vi "esp32.vi"() -> ()   [LabVIEW 2017]
panel:
  out "parameter value":string
  out "function value":string
  in  "stop 4":bool
  out "NewVal":enum16{"input", "output", "disable"}(ring)
  out "appended array":refnum<vi>[](array[refnum])
  out "bytes written 4":i32
  out "bytes written 2":i32
  in  "stop 3":bool
  in  "Tab Control":T1(tab)
  in  "address":string="10.5.4.109"
  in  "Port":u16=8888
  in  "pin 14":enum16{"input", "output", "disable"}(ring)=enum."disable"
  in  "VIN":enum16{""}(ring)
  in  "GND 2":enum16{""}(ring)
  in  "3.3 V":enum16{""}(ring)
  in  "GND":enum16{""}(ring)
  in  "pin 15":enum16{"input", "output", "disable"}(ring)=enum."disable"
  in  "pin 02":enum16{"input", "output", "disable"}(ring)=enum."disable"
  in  "pin 04":enum16{"input", "output", "disable"}(ring)=enum."disable"
  in  "pin 16":enum16{"input", "output", "disable"}(ring)=enum."disable"
  in  "pin 17":enum16{"input", "output", "disable"}(ring)=enum."disable"
  in  "pin 05":enum16{"input", "output", "disable"}(ring)=enum."disable"
  in  "pin 18":enum16{"input", "output", "disable"}(ring)=enum."disable"
  in  "pin 19":enum16{"input", "output", "disable"}(ring)=enum."disable"
  in  "pin 21":enum16{"input", "output", "disable"}(ring)=enum."disable"
  in  "pin 03":enum16{"input", "output", "disable"}(ring)=enum."disable"
  in  "pin 01":enum16{"input", "output", "disable"}(ring)=enum."disable"
  in  "pin 22":enum16{"input", "output", "disable"}(ring)=enum."disable"
  in  "pin 23":enum16{"input", "output", "disable"}(ring)=enum."disable"
  in  "pin 12":enum16{"input", "output", "disable"}(ring)=enum."disable"
  in  "pin 27":enum16{"input", "output", "disable"}(ring)=enum."disable"
  in  "pin 26":enum16{"input", "output", "disable"}(ring)=enum."disable"
  in  "pin 25":enum16{"input", "output", "disable"}(ring)=enum."disable"
  in  "pin 33":enum16{"input", "output", "disable"}(ring)=enum."disable"
  in  "pin 32":enum16{"input", "output", "disable"}(ring)=enum."disable"
  in  "pin 35":enum16{"input", "output", "disable"}(ring)=enum."disable"
  in  "pin 34":enum16{"input", "output", "disable"}(ring)=enum."disable"
  in  "pin 39":enum16{"input", "output", "disable"}(ring)=enum."disable"
  in  "pin 36":enum16{"input", "output", "disable"}(ring)=enum."disable"
  in  "EN":enum16{""}(ring)
  in  "pin 13":enum16{"disable", "input", "output"}(ring)
  in  "output 36":bool
  out "input 36":bool
  in  "output 39":bool
  out "input 39":bool
  in  "output 12":bool
  in  "output 15":bool
  out "input 15":bool
  in  "output 2":bool
  out "input 2":bool
  in  "output 4":bool
  out "input 4":bool
  in  "output 16":bool
  out "input 16":bool
  in  "output 17":bool
  out "input 17":bool
  in  "output 5":bool
  out "input 5":bool
  in  "output 18":bool
  out "input 18":bool
  in  "output 19":bool
  out "input 19":bool
  in  "output 21":bool
  out "input 21":bool
  in  "output 3":bool
  out "input 3":bool
  in  "output 1":bool
  out "input 1":bool
  in  "output 22":bool
  out "input 22":bool
  in  "output 23":bool
  out "input 23":bool
  in  "output 34":bool
  out "input 34":bool
  out "input 13":bool
  in  "output 35":bool
  out "input 35":bool
  in  "output 32":bool
  out "input 32":bool
  in  "output 33":bool
  out "input 33":bool
  in  "output 25":bool
  out "input 25":bool
  in  "output 26":bool
  out "input 26":bool
  in  "output 27":bool
  out "input 27":bool
  in  "output 14":bool
  out "input 14":bool
  in  "output 13":bool
  out "input 12":bool
  in  "data in":string
  in  "Send Button":bool
  in  "stop 2":bool
  out "bytes written 3":i32
  out "data out":string
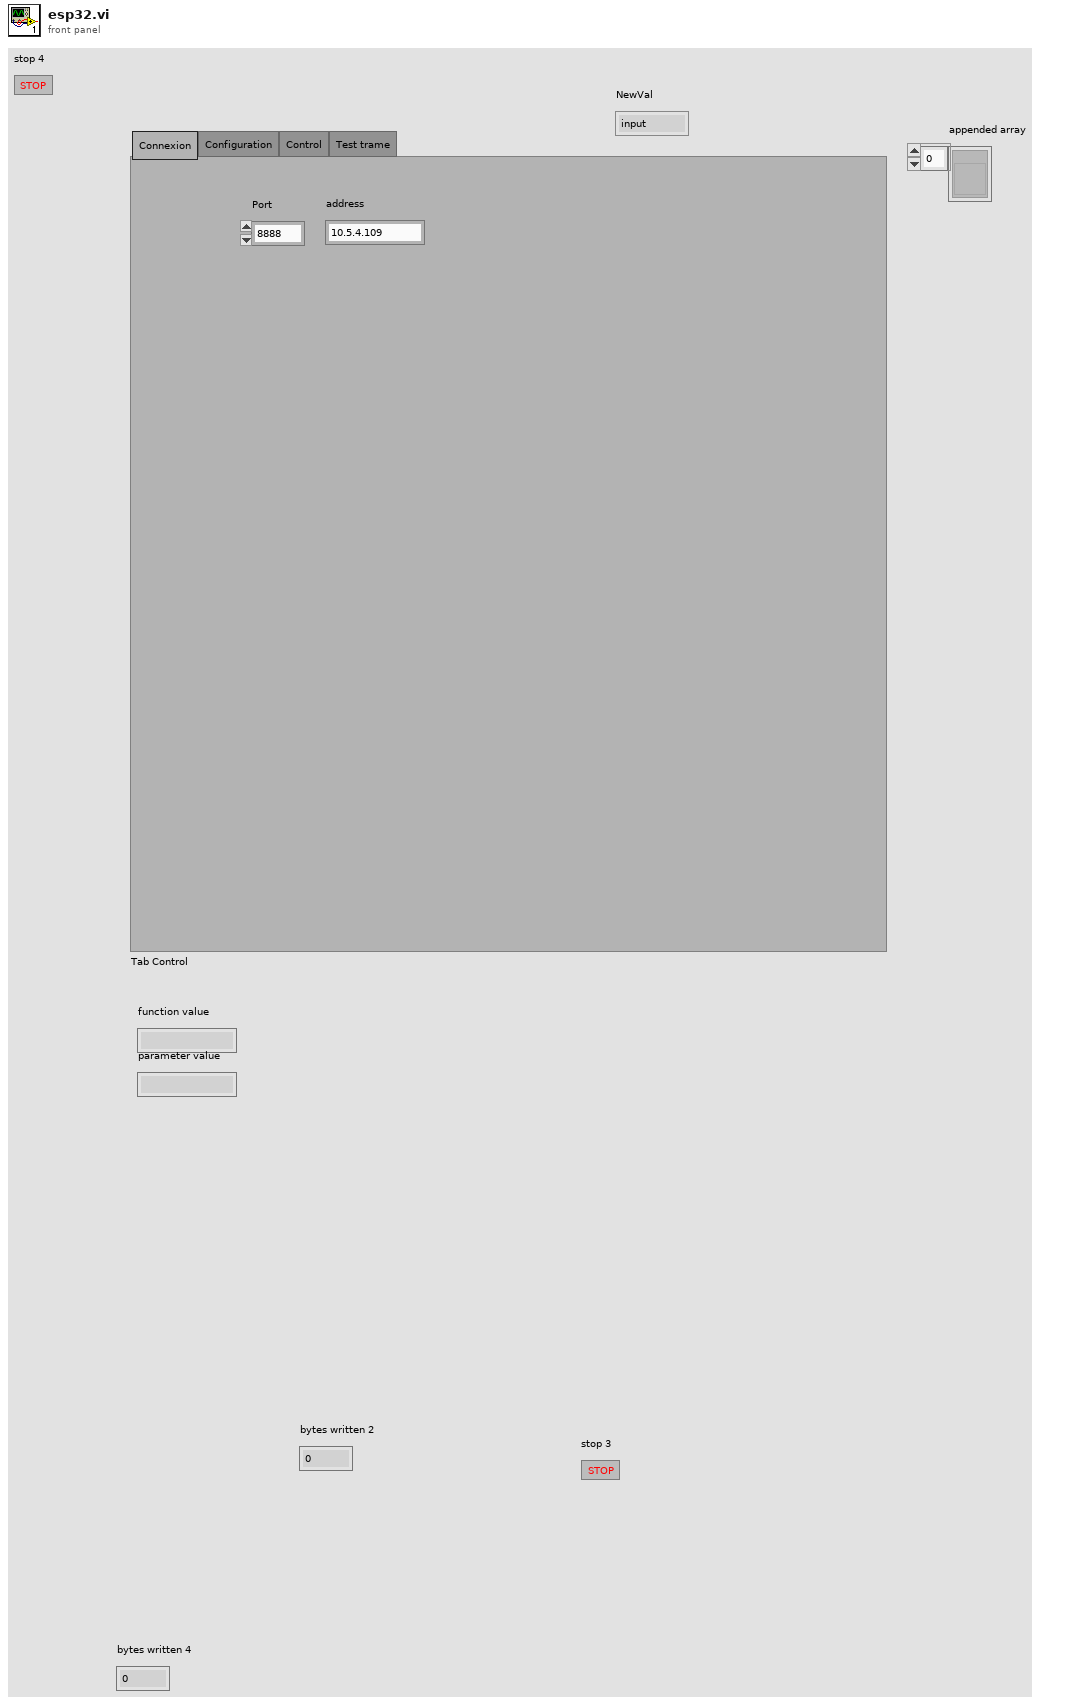
[diagram p1: front panel]
types:
  T1 = enum32{"Connexion", "Configuration", "Control", "Test trame"}
  T2 = enum16{"Standard", "Buffered", "CRLF", "Immediate"}
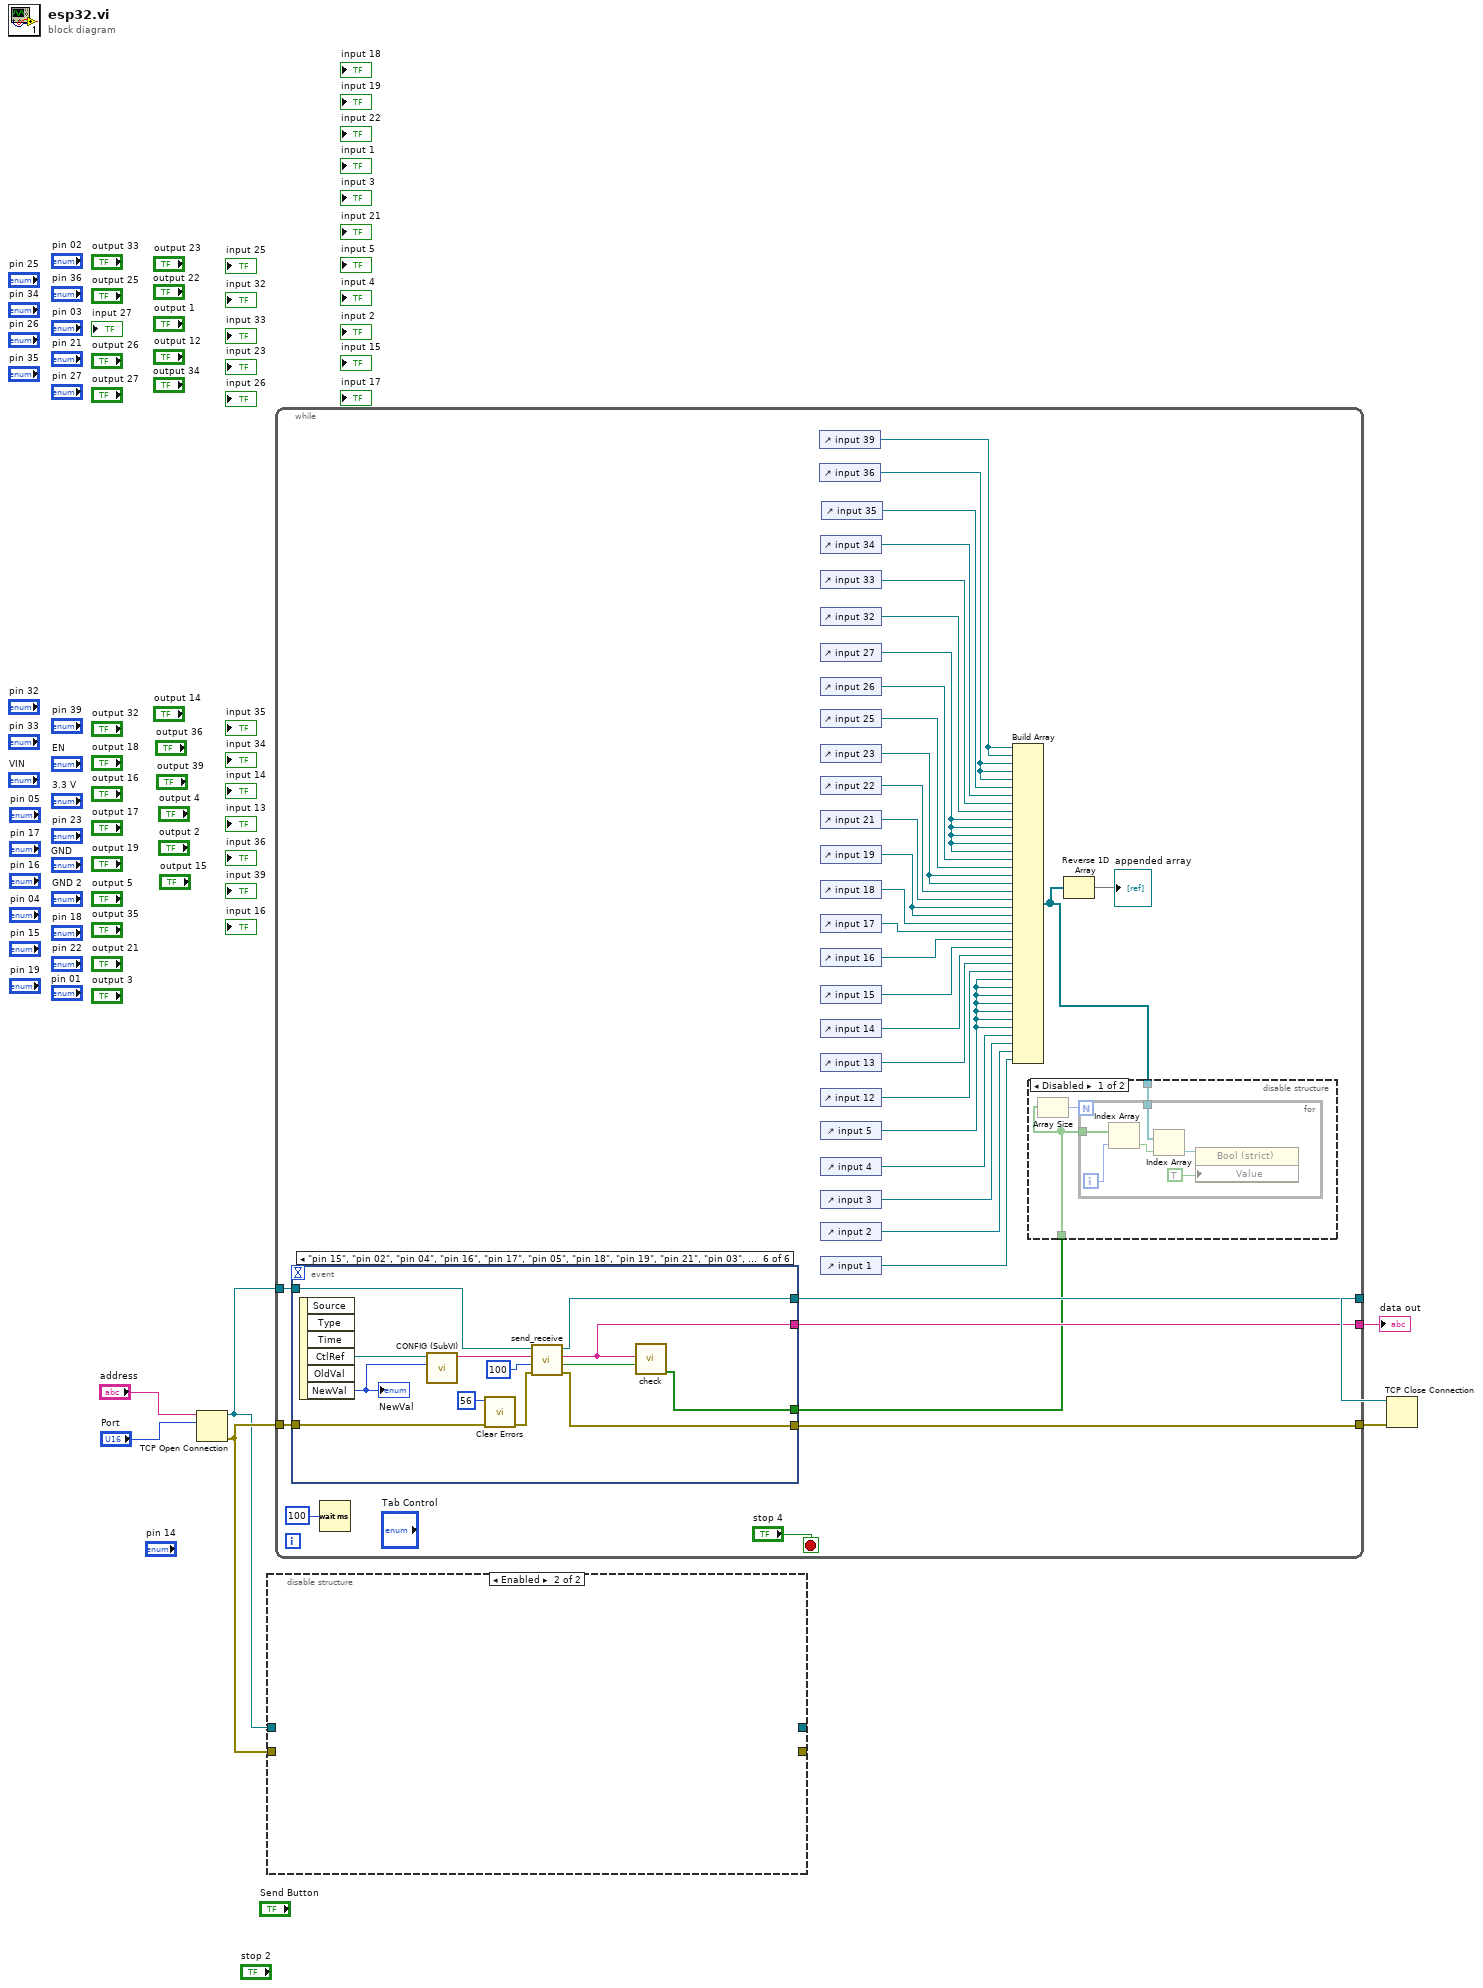
[diagram p0: block diagram]
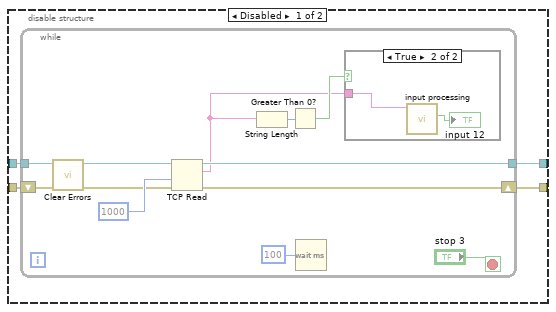
[diagram p2: hidden frame]
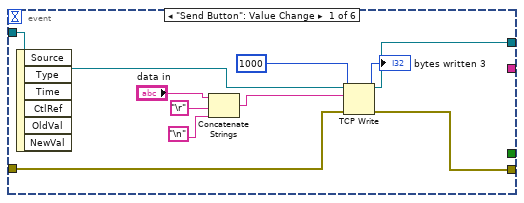
[diagram p5: hidden frame]
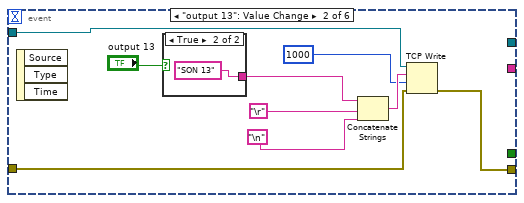
[diagram p6: hidden frame]
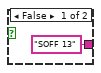
[diagram p7: hidden frame]
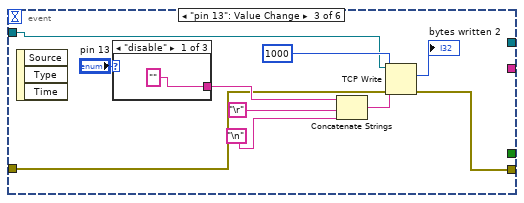
[diagram p8: hidden frame]
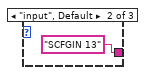
[diagram p9: hidden frame]
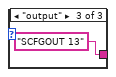
[diagram p10: hidden frame]
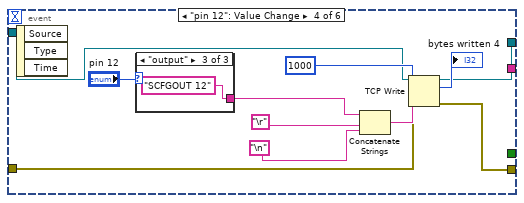
[diagram p11: hidden frame]
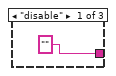
[diagram p12: hidden frame]
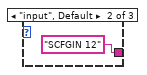
[diagram p13: hidden frame]
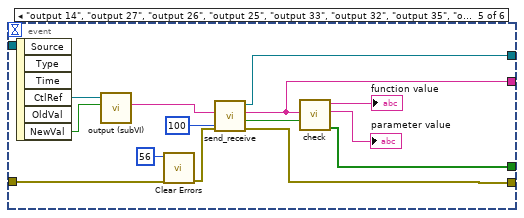
[diagram p14: hidden frame]
diagram:
  n1 = TCP Open Connection(address="address", remote port or service name="Port") -> (connection ID=w4:refnum<k5>, error out=w5:errorcluster)  [unwired: 3 in]
  n2 = disable-structure shown="Enabled" {
    disable-tunnel: w5 -> [w11 _]
    disable-tunnel: w4 -> [w10 _]
    disable-tunnel: [w9 _] -> _
    disable-tunnel: [w8 _] -> _
    frame Disabled {
      n3 = while {
        tunnel: w10 -> [w24]
        shift-right: [w22] -> w9
        shift-left: w11 -> [w18]
        tunnel: [w21] -> w8
        stop <- "stop 3" stop-if-true
        n4 = call <vilib>:"Clear Errors.vi"("error in (no error)"=w18) -> ("error out"=w17:errorcluster)  [unwired: 5 in, 1 out]
        n5 = TCP Read(connection ID=w24, error in (no error)=w17, 9:1000 ("timeout ms (25000)")) -> (bytes to read=w13:i32, connection ID out=w21:refnum<k5>, data out=w14:string, error out=w22:errorcluster, 7:w12:T2)
        n6 = String Length(string=w14) -> (length=w16:i32)
        n7 = Greater Than 0?(x=w16) -> (x > 0?=w15:bool)
        n8 = Wait (ms)(milliseconds to wait=u32 100) -> ()  [unwired: 1 out]
        n9 = case shown="True" w15 {
          tunnel: w14 -> [_ w25]
          frame False {
          }
          frame True {
            n10 = call "input processing.vi"("String"=w25) -> ("inputan 5"=→"input 12":bool)  [unwired: 9 in, 1 out]
          }
        }
      }
    }
    frame Enabled {
    }
  }
  n11 = while {
    tunnel: w5 -> [w60]
    tunnel: [w58] -> w2
    tunnel: w4 -> [w61]
    tunnel: [w57] -> w1
    tunnel: [w55] -> w3
    stop <- "stop 4" stop-if-true
    n12 = event shown="[5] \"pin 15\", \"pin 02\", \"pin 04\", \"pin 16\", \"pin 17\", \"pin 05\", \"pin 18\", \"pin 19\", \"pin 21\", \"pin 03\", \"pin 01\", \"pin 22\", \"pin 23\", \"pin 27\", \"pin 26\", \"pin 25\", \"pin 33\", \"pin 32\", \"pin 35\", \"pin 34\", \"pin 39\", \"pin 36\", \"pin 14\": Value Change" {
      selector: _ -> [_ _ _ _ _ _]
      dyn-events: _ -> [_ _ _ _ _ _]
      timeout: _ -> [_ _ _ _ _ _]
      tunnel: w61 -> [w73 w81 w92 w106 _ w142]
      tunnel: w60 -> [w75 w82 w93 w107 w127 w137]
      tunnel: [w74 w84 w94 w108 w128 w138] -> w58
      tunnel: [w72 _ _ w105 w123 w139] -> w57
      tunnel: [_ _ _ _ w122 w134] -> w55
      tunnel: [_ _ _ _ w119 w133] -> w27
      event "Send Button": Value Change {
        n13 = event-data() -> ()  [unwired: 1 in, 6 out]
        n14 = Concatenate Strings("data in", "\r", "\n") -> (w80:string)
        n15 = TCP Write(connection ID=w73, data in=w80, error in (no error)=w75, 9:1000 ("timeout ms (25000)")) -> (connection ID out=w72:refnum<k5>, bytes written=→"bytes written 3":i32, error out=w74:errorcluster)
      }
      event "output 13": Value Change {
        n16 = event-data() -> ()  [unwired: 1 in, 3 out]
        n17 = case shown="True" "output 13" {
          tunnel: ["SOFF 13" "SON 13"] -> w83
          frame False {
          }
          frame True {
          }
        }
        n18 = Concatenate Strings(w83, "\r", "\n") -> (w88:string)
        n19 = TCP Write(connection ID=w81, data in=w88, error in (no error)=w82, 9:1000 ("timeout ms (25000)")) -> (error out=w84:errorcluster)  [unwired: 2 out]
      }
      event "pin 13": Value Change {
        n20 = event-data() -> ()  [unwired: 1 in, 3 out]
        n21 = case shown="\"disable\"" "pin 13" {
          tunnel: ["" "SCFGIN 13" "SCFGOUT 13"] -> w95
          frame "disable" {
          }
          frame "input", Default {
          }
          frame "output" {
          }
        }
        n22 = Concatenate Strings(w95, "\r", "\n") -> (w100:string)
        n23 = TCP Write(connection ID=w92, data in=w100, error in (no error)=w93, 9:1000 ("timeout ms (25000)")) -> (bytes written=→"bytes written 2":i32, error out=w94:errorcluster)  [unwired: 1 out]
      }
      event "pin 12": Value Change {
        n24 = event-data() -> ()  [unwired: 1 in, 3 out]
        n25 = case shown="\"output\"" "pin 12" {
          tunnel: ["" "SCFGIN 12" "SCFGOUT 12"] -> w110
          frame "disable" {
          }
          frame "input", Default {
          }
          frame "output" {
          }
        }
        n26 = Concatenate Strings(w110, "\r", "\n") -> (w115:string)
        n27 = TCP Write(connection ID=w106, data in=w115, error in (no error)=w107, 9:1000 ("timeout ms (25000)")) -> (connection ID out=w105:refnum<k5>, bytes written=→"bytes written 4":i32, error out=w108:errorcluster)
      }
      event "output 14", "output 27", "output 26", "output 25", "output 33", "output 32", "output 35", "output 34", "output 23", "output 22", "output 1", "output 3", "output 21", "output 19", "output 18", "output 5", "output 17", "output 16", "output 4", "output 2", "output 15", "output 12", "output 39", "output 36": Value Change {
        n28 = event-data() -> ("CtlRef"=w125:refnum<vi>, "NewVal"=w126:bool)  [unwired: 1 in, 4 out]
        n29 = call "output (subVI).vi"("NewVal in"=w126, "Boolean in"=w125) -> ("string out"=w124:string)  [unwired: 9 in]
        n30 = call <vilib>:"Clear Errors.vi"("error in (no error)"=w127, "specific error code to clear (0: all)"=56) -> ("error out"=w130:errorcluster)  [unwired: 4 in, 1 out]
        n31 = call "send_receive.vi"("error in (no error)"=w130, "time"=u32 100, "data in"=w124) -> ("error out"=w128:errorcluster, "Result"=w132:bool, "data out"=w122:string, "connection ID out"=w123:refnum<k5>)  [unwired: 5 in]
        n32 = call "check.vi"("input result"=w132, "input string"=w122) -> ("Array"=w119:bool[], "parameter value"=→"parameter value":string, "function value"=→"function value":string)  [unwired: 6 in, 1 out]
      }
      event "pin 15", "pin 02", "pin 04", "pin 16", "pin 17", "pin 05", "pin 18", "pin 19", "pin 21", "pin 03", "pin 01", "pin 22", "pin 23", "pin 27", "pin 26", "pin 25", "pin 33", "pin 32", "pin 35", "pin 34", "pin 39", "pin 36", "pin 14": Value Change {
        n33 = event-data() -> ("CtlRef"=w145:refnum<vi>, "NewVal"=w144:enum16{"input", "output", "disable"})  [unwired: 1 in, 4 out]
        "NewVal" <- w144
        n34 = call "CONFIG (SubVI).vi"("NewVal"=w144, "Enum in"=w145) -> ("String"=w143:string)  [unwired: 9 in]
        n35 = call <vilib>:"Clear Errors.vi"("error in (no error)"=w137, "specific error code to clear (0: all)"=56) -> ("error out"=w136:errorcluster)  [unwired: 4 in, 1 out]
        n36 = call "send_receive.vi"("error in (no error)"=w136, "time"=u32 100, "data in"=w143, "connection ID in"=w142) -> ("error out"=w138:errorcluster, "Result"=w141:bool, "data out"=w134:string, "connection ID out"=w139:refnum<k5>)  [unwired: 4 in]
        n37 = call "check.vi"("input result"=w141, "input string"=w134) -> ("Array"=w133:bool[])  [unwired: 6 in, 3 out]
      }
    }
    n38 = Wait (ms)(milliseconds to wait=u32 100) -> ()  [unwired: 1 out]
    n39 = control-ref of="input 39"() -> (w53:refnum<vi>)
    n40 = control-ref of="input 36"() -> (w52:refnum<vi>)
    n41 = control-ref of="input 34"() -> (w50:refnum<vi>)
    n42 = control-ref of="input 33"() -> (w49:refnum<vi>)
    n43 = control-ref of="input 32"() -> (w48:refnum<vi>)
    n44 = control-ref of="input 27"() -> (w47:refnum<vi>)
    n45 = control-ref of="input 26"() -> (w46:refnum<vi>)
    n46 = control-ref of="input 25"() -> (w45:refnum<vi>)
    n47 = control-ref of="input 23"() -> (w44:refnum<vi>)
    n48 = control-ref of="input 22"() -> (w43:refnum<vi>)
    n49 = control-ref of="input 21"() -> (w42:refnum<vi>)
    n50 = control-ref of="input 19"() -> (w41:refnum<vi>)
    n51 = control-ref of="input 18"() -> (w40:refnum<vi>)
    n52 = control-ref of="input 17"() -> (w39:refnum<vi>)
    n53 = control-ref of="input 16"() -> (w38:refnum<vi>)
    n54 = control-ref of="input 15"() -> (w37:refnum<vi>)
    n55 = control-ref of="input 14"() -> (w36:refnum<vi>)
    n56 = control-ref of="input 13"() -> (w35:refnum<vi>)
    n57 = control-ref of="input 12"() -> (w34:refnum<vi>)
    n58 = control-ref of="input 5"() -> (w33:refnum<vi>)
    n59 = control-ref of="input 4"() -> (w31:refnum<vi>)
    n60 = control-ref of="input 3"() -> (w30:refnum<vi>)
    n61 = control-ref of="input 2"() -> (w29:refnum<vi>)
    n62 = control-ref of="input 1"() -> (w32:refnum<vi>)
    n63 = control-ref of="input 35"() -> (w51:refnum<vi>)
    n64 = Build Array(w53, w53, w52, w52, w52, w51, w50, w49, w48, w47, w47, w47, w47, w47, w46, w45, w44, w44, w43, w42, w41, w41, w40, w39, w38, w37, w36, w35, w34, w33, w33, w33, w33, w33, w33, w33, w31, w30, w29, w32) -> (w28:refnum<vi>[])
    n65 = disable-structure shown="Disabled" {
      disable-tunnel: w28 -> [w64 _]
      disable-tunnel: w27 -> [w62 _]
      frame Disabled {
        n66 = Array Size(array=w62) -> (size(s)=w63:i32)
        n67 = for {
          N: w63 -> [_]
          tunnel: w62 -> [w70]
          tunnel: w64 -> [w67]
          i -> [w69]
          n68 = Index Array(array=w70, index=w69) -> (element=w66:bool)
          n69 = Index Array(array=w67, index=w66) -> (element=w68:refnum<vi>)
          n70 = property class="Bool (strict)"(reference=w68, "Value"=TRUE) -> ()  [unwired: 1 in, 2 out]
        }
      }
      frame Enabled {
      }
    }
    n71 = Reverse 1D Array(array=w28) -> (reversed array=→"appended array":refnum<vi>[])
  }
  "data out" <- w3
  n72 = TCP Close Connection(connection ID=w1, error in (no error)=w2) -> ()  [unwired: 1 in, 2 out]
